vi "VI Tree.vi"   [LabVIEW 2009, in "CAEN PSM.lvlib"]
doc: "This is the instrument driver for the CAEN N14XX. The VI Tree displays all the user-callable VIs of the instrument driver in an organized table."
uses:
  <instrlib>/CAEN PSM/CAEN PSM.lvlib
panel:
  # "(c) 2012 CAEN SpA.  ALL RIGHTS RESERVED."
  # "SEE DIAGRAM\nFOR VI TREE."
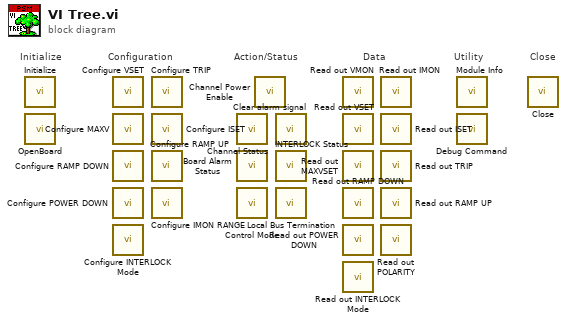
[diagram p0: block diagram]
diagram:
  # "Configuration"
  # "Utility"
  # "Data"
  # "Action/Status"
  # "Close"
  # "Initialize"
  n1 = call <instrlib>:"Initialize.vi"() -> ()  [unwired: 10 in, 2 out]
  n2 = call <instrlib>:"OpenBoard.vi"() -> ()  [unwired: 10 in, 2 out]
  n3 = call <instrlib>:"Configure VSET.vi"() -> ()  [unwired: 10 in, 2 out]
  n4 = call <instrlib>:"Configure MAXV.vi"() -> ()  [unwired: 10 in, 2 out]
  n5 = call <instrlib>:"Configure RAMP DOWN.vi"() -> ()  [unwired: 10 in, 2 out]
  n6 = call <instrlib>:"Configure POWER DOWN.vi"() -> ()  [unwired: 10 in, 2 out]
  n7 = call <instrlib>:"Configure INTERLOCK Mode.vi"() -> ()  [unwired: 10 in, 2 out]
  n8 = call <instrlib>:"Configure TRIP.vi"() -> ()  [unwired: 10 in, 2 out]
  n9 = call <instrlib>:"Configure ISET.vi"() -> ()  [unwired: 10 in, 2 out]
  n10 = call <instrlib>:"Configure RAMP UP.vi"() -> ()  [unwired: 10 in, 2 out]
  n11 = call <instrlib>:"Configure IMON RANGE.vi"() -> ()  [unwired: 10 in, 2 out]
  n12 = call <instrlib>:"Channel Status.vi"() -> ()  [unwired: 9 in, 3 out]
  n13 = call <instrlib>:"Board Alarm Status.vi"() -> ()  [unwired: 8 in, 4 out]
  n14 = call <instrlib>:"Control Mode.vi"() -> ()  [unwired: 8 in, 4 out]
  n15 = call <instrlib>:"Channel Power Enable.vi"() -> ()  [unwired: 10 in, 2 out]
  n16 = call <instrlib>:"Clear alarm signal.vi"() -> ()  [unwired: 10 in, 2 out]
  n17 = call <instrlib>:"INTERLOCK Status.vi"() -> ()  [unwired: 9 in, 3 out]
  n18 = call <instrlib>:"Local Bus Termination.vi"() -> ()  [unwired: 9 in, 3 out]
  n19 = call <instrlib>:"Read out VMON.vi"() -> ()  [unwired: 9 in, 3 out]
  n20 = call <instrlib>:"Read out VSET.vi"() -> ()  [unwired: 8 in, 4 out]
  n21 = call <instrlib>:"Read out MAXVSET.vi"() -> ()  [unwired: 8 in, 4 out]
  n22 = call <instrlib>:"Read out RAMP DOWN.vi"() -> ()  [unwired: 8 in, 4 out]
  n23 = call <instrlib>:"Read out POWER DOWN.vi"() -> ()  [unwired: 9 in, 3 out]
  n24 = call <instrlib>:"Read out INTERLOCK Mode.vi"() -> ()  [unwired: 9 in, 3 out]
  n25 = call <instrlib>:"Read out IMON.vi"() -> ()  [unwired: 8 in, 4 out]
  n26 = call <instrlib>:"Read out ISET.vi"() -> ()  [unwired: 8 in, 4 out]
  n27 = call <instrlib>:"Read out TRIP.vi"() -> ()  [unwired: 8 in, 4 out]
  n28 = call <instrlib>:"Read out RAMP UP.vi"() -> ()  [unwired: 8 in, 4 out]
  n29 = call <instrlib>:"Read out POLARITY.vi"() -> ()  [unwired: 9 in, 3 out]
  n30 = call <instrlib>:"Module Info.vi"() -> ()  [unwired: 9 in, 3 out]
  n31 = call <instrlib>:"Debug Command.vi"() -> ()  [unwired: 11 in, 5 out]
  n32 = call <instrlib>:"Close.vi"() -> ()  [unwired: 11 in, 1 out]
